vi "test - Fit Controls to Rect.vi"() -> ()   [LabVIEW 2017]
uses:
  <vilib>/Utility/miscctls.llb/LVRectTypeDef.ctl
panel:
  in  "Enum":enum16{"1", "2", "3"}(ring)
  out "Rect pane":T1
  out "Rect":T1
  in  "Ring":u16(ring)
  in  "Boolean 2":bool
  in  "Boolean":bool
  in  "String":string
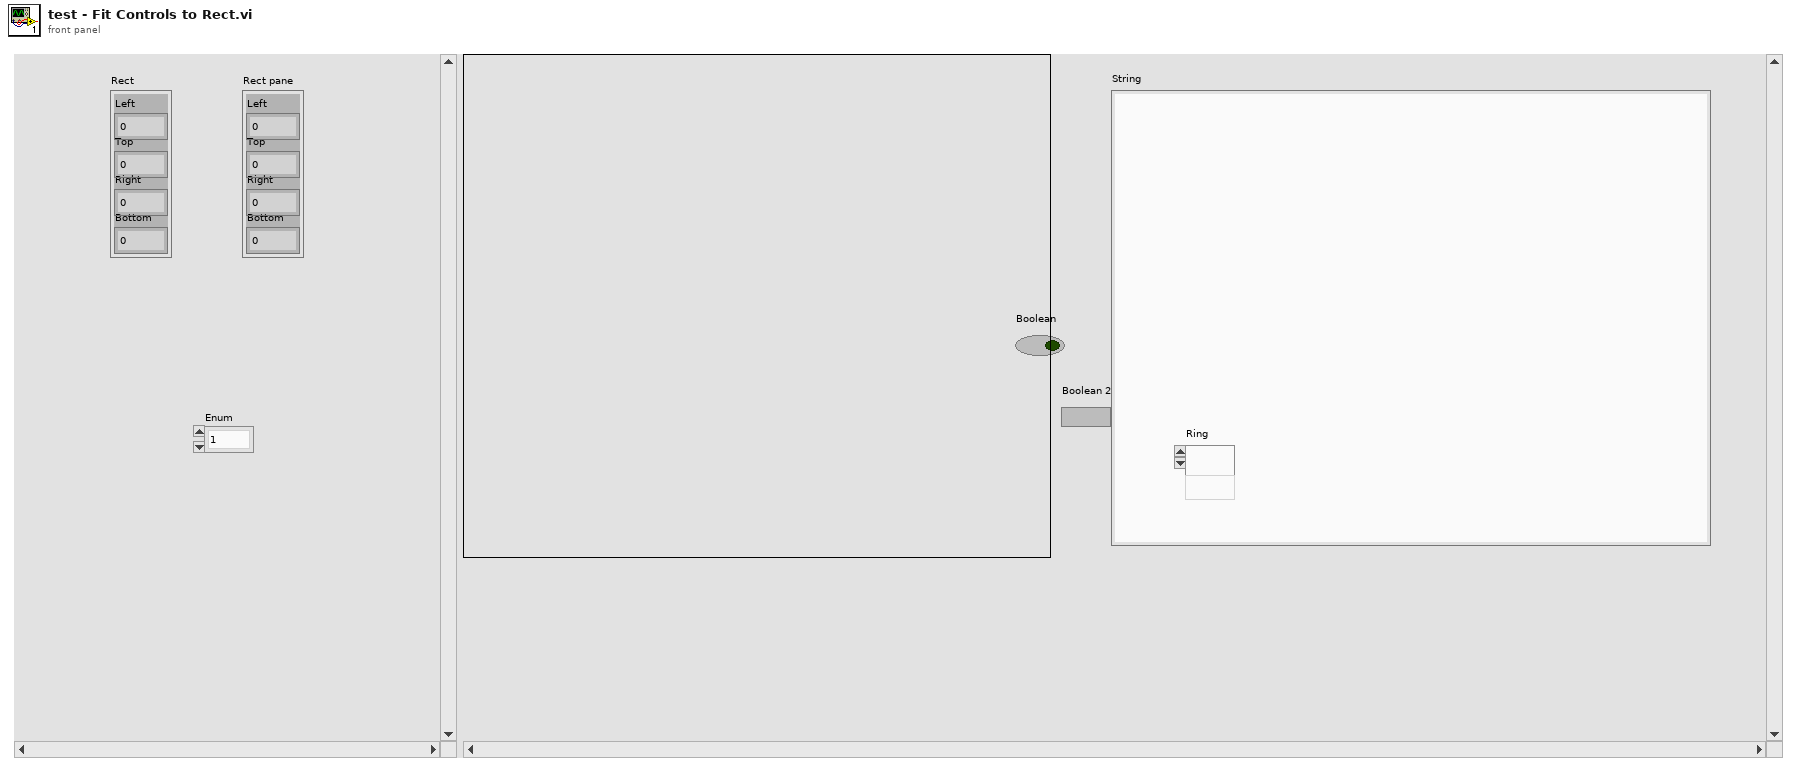
[diagram p1: front panel]
types:
  T1 = typedef "LVRectTypeDef.ctl" = cluster{"Left":i16, "Top":i16, "Right":i16, "Bottom":i16}
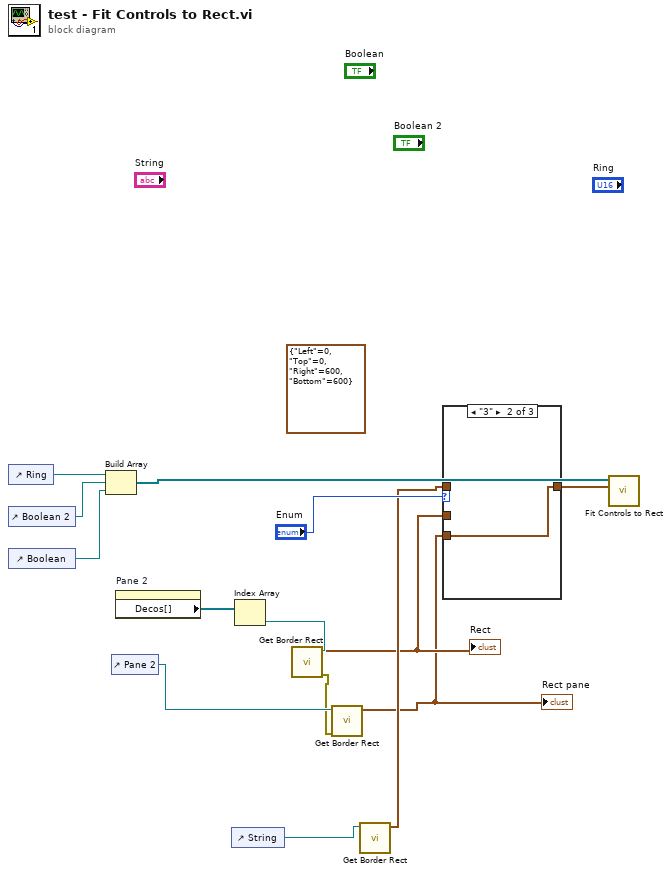
[diagram p0: block diagram]
diagram:
  (unwired) T1 {"Left"=0, "Top"=0, "Right"=600, "Bottom"=600} ("Rect")
  n1 = control-ref of="Ring"() -> (w14:refnum<vi>)
  n2 = control-ref of="Boolean 2"() -> (w13:refnum<vi>)
  n3 = control-ref of="Boolean"() -> (w12:refnum<vi>)
  n4 = Build Array(w14, w13, w12) -> (w11:refnum<vi>[])
  n5 = control-ref of="Pane 2"() -> (w8:refnum<vi>)
  n6 = property on="Pane 2" class="Pane"() -> ("Decos[]"=w10:refnum<vi>[])  [unwired: 2 in, 2 out]
  n7 = control-ref of="String"() -> (w6:refnum<vi>)
  n8 = Index Array(array=w10) -> (element=w9:refnum<vi>)  [unwired: 1 in]
  n9 = call "Get Border Rect.vi"("borderObj Ref"=w9) -> ("Error out"=w7:errorcluster, "Rect"=w2:T1)  [unwired: 9 in]
  "Rect" <- w2
  n10 = call "Get Border Rect.vi"("Error in"=w7, "borderObj Ref"=w8) -> ("Rect"=w1:T1)  [unwired: 8 in, 1 out]
  "Rect pane" <- w1
  n11 = call "Get Border Rect.vi"("borderObj Ref"=w6) -> ("Rect"=w4:T1)  [unwired: 9 in, 1 out]
  n12 = case shown="\"3\"" "Enum" {
    tunnel: w4 -> [_ _ w17]
    tunnel: [w15 w16 w17] -> w3
    tunnel: w2 -> [w15 _ _]
    tunnel: w1 -> [_ w16 _]
    frame "1", Default {
    }
    frame "3" {
    }
    frame "2" {
    }
  }
  n13 = call "Fit Controls to Rect.vi"("Rect"=w3, "GObjs"=w11) -> ()  [unwired: 4 in, 2 out]
